vi "module discover And Connect.vi"(7 "dll path in":path, 8 "error in (no error)":errorcluster, 9 "transport":i32, 10 "result":cluster{"value":i32, "error":i32}, 11 "id":u32) -> (0 "error out":errorcluster, 2 "result out":cluster{"value":i32, "error":i32}, 3 "id out":u32)   [LabVIEW 2025]
doc: "aLIBEXPORT void __stdcall module_discoverAndConnect(\n unsigned int* id, \n struct Result* result, \n int transport = (int)USB);"
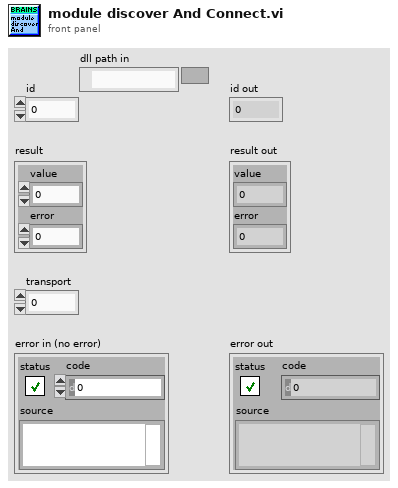
[diagram p1: front panel]
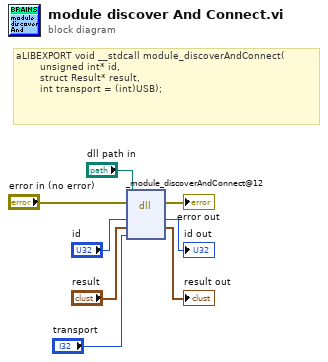
[diagram p0: block diagram]
diagram:
  # "aLIBEXPORT void __stdcall module_discoverAndConnect(\n        unsigned int* id, \n        struct Result* result, \n        int transport = (int)USB);"
  n1 = dll-call lib="?" fn="_module_discoverAndConnect@12"(path in="dll path in", error in="error in (no error)", "id"="id", "result"="result", "transport"="transport") -> (error out=→"error out":errorcluster, "id"=→"id out":u32, "result"=→"result out":cluster{"value":i32, "error":i32})  [unwired: 3 in, 1 out]
